vi "create client connector.vi"(8 "error in":errorcluster, 11 "engine pointer":u64) -> (0 "error out":errorcluster, 3 "client connector out":refnum<class "client connector.lvclass">)   [LabVIEW 2016, in "client connector.lvclass"]
uses:
  client connector.lvclass
  C:/Users/IEUser/Desktop/libasynclvtls/tls classes/connection creator/connection creator.lvclass
  dllwrapper/library path.vi
  dllwrapper/async tls dl.lvlib
  connection creator.lvclass
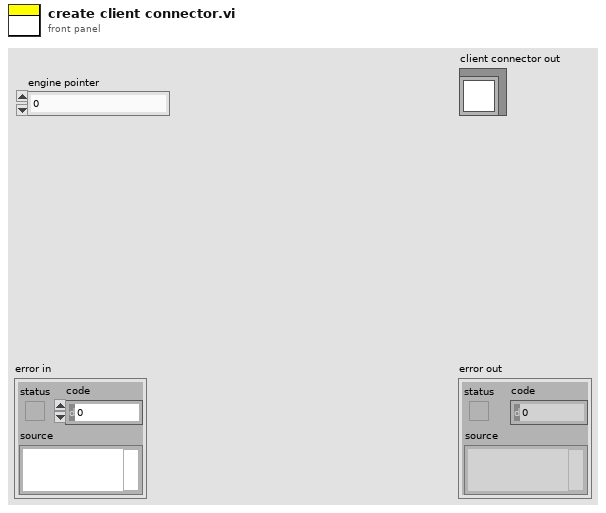
[diagram p1: front panel]
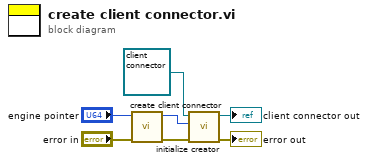
[diagram p0: block diagram]
diagram:
  n1 = call "create client connector.vi"("error in"="error in", "engine"="engine pointer") -> ("error out"=w7:errorcluster, "client out"=w2:u64)  [unwired: 8 in]
  n2 = call "initialize creator.vi"("error in"=w7, "pointer"=w2, "connection creator in"=refnum<class "client connector.lvclass"> refnum ("client connector.lvclass")) -> ("error out"=→"error out":errorcluster, "connection creator out"=→"client connector out":refnum<class "client connector.lvclass">)  [unwired: 7 in]
